vi "Cleanup.vi"(8 "error in (no error)":errorcluster, 11 "LV Client in":refnum<class "LV Client.lvclass">) -> (0 "error out":errorcluster)   [LabVIEW 2020, in "LV Client.lvclass"]
uses:
  LV Client.lvclass
  lv-msg-simple/Stream-Simple-Msg/Manager/Manager.lvclass
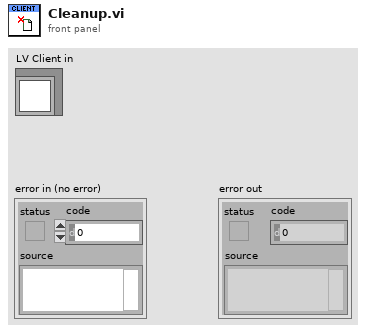
[diagram p1: front panel]
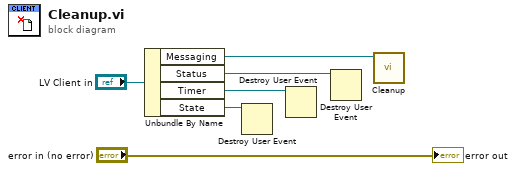
[diagram p0: block diagram]
diagram:
  n1 = Unbundle By Name("LV Client in") -> ("Messaging"=w4:refnum<class "Manager.lvclass">, "Status"=w1:refnum<user-event>, "Timer"=w2:refnum<user-event>, "State"=w3:refnum<user-event>)
  n2 = Destroy User Event(user event=w3) -> ()  [unwired: 1 in, 1 out]
  n3 = Destroy User Event(user event=w2) -> ()  [unwired: 1 in, 1 out]
  n4 = Destroy User Event(user event=w1) -> ()  [unwired: 1 in, 1 out]
  n5 = call "Cleanup.vi"("Manager in"=w4) -> ()  [unwired: 10 in, 1 out]
  "error out" <- "error in (no error)"
